vi "Tests_ping.vi"() -> ()   [LabVIEW 2019]
uses:
  <vilib>/Platform/TimedLoop/XDataNode/timing_clust.ctl
  <vilib>/Platform/TimedLoop/XDataNode/nitl_modes.ctl
  <vilib>/Platform/TimedLoop/XDataNode/wakeup.ctl
  <vilib>/Utility/file.llb/Read Delimited Spreadsheet (string).vi
  <vilib>/Platform/TimedLoop/XDataNode/XDataNode.xnode
  <vilib>/Platform/TimedLoop/XDataNode/XDNodeRunTimeDep.lvlib
panel:
  in  "Bouton OK":bool
  out "Booléen":bool
  in  "stop":bool
  out "Systèmes inatteignable":string[][](array[string])
  out "Status":i32(ring) items=["Success"=0, "DestinationNetworkUnreachable"=11002, "DestinationHostUnreachable"=11003, "DestinationProhibited, DestinationProtocolUnreachable"=11004, "DestinationPortUnreachable"=11005, "NoResources"=11006, "BadOption"=11007, "HardwareError"=11008, "PacketTooBig"=11009, "TimedOut"=11010, "BadRoute"=11012, "TtlExpired"=11013, "TtlReassemblyTimeExceeded"=11014, "ParameterProblem"=11015, "SourceQuench"=11016, "BadDestination"=11018, "DestinationUnreachable"=11040, "TimeExceeded"=11041, "BadHeader"=11042, "UnrecognizedNextHeader"=11043, "IcmpError"=11044, "DestinationScopeMismatch"=11045, "Unknown"=-1]
  out "all rows":string[][](array[string]) caption="toutes les lignes"
  # "Tests réseau"
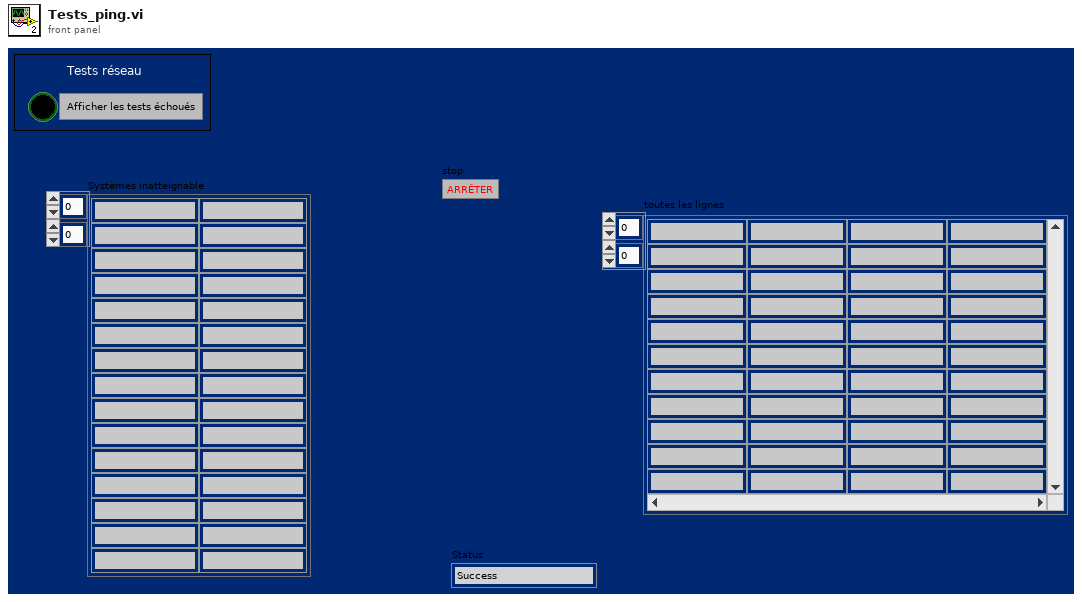
[diagram p1: front panel]
types:
  T1 = typedef "XDNodeRunTimeDep.lvlib/timing_clust.ctl" = cluster{"Expected End [f-1]":u64, "Actual End [f-1]":u64, "Finished Late? [f-1]":bool, "Expected End [i-1]":u64, "Actual End [i-1]":u64, "Finished Late? [i-1]":bool, "Expected Start [i]":u64, "Actual Start [i]":u64, "Expected Start [f]":u64, "Actual Start [f]":u64, "Source Name":string, "Structure Name":string, "Period":i64, "Deadline":i64, "Offset":i64, "Start":i64, "Priority":i32, "Timeout":i32, "Mode":T2, "Wakeup Reason":T3, "Error":errorcluster, "Source Type":string, "Secondary Source Type":string, "Global End Time":u64, "Global Start Time":u64, "Frame Duration":u64, "Iteration Duration":u64, "Assigned CPU":i32, "I/O Scan Engine Mode":u32}
  T2 = typedef "XDNodeRunTimeDep.lvlib/nitl_modes.ctl" = enum32{"No Change", "Process missed periods, maintain original phase", "Discard missed periods, maintain original phase", "Process missed periods, ignore original phase", "Discard missed periods, ignore original phase"}
  T3 = typedef "XDNodeRunTimeDep.lvlib/wakeup.ctl" = enum32{"Normal", "Aborted", "Asynchronous wakeup", "Timing source error", "Timed loop error", "Timeout"}
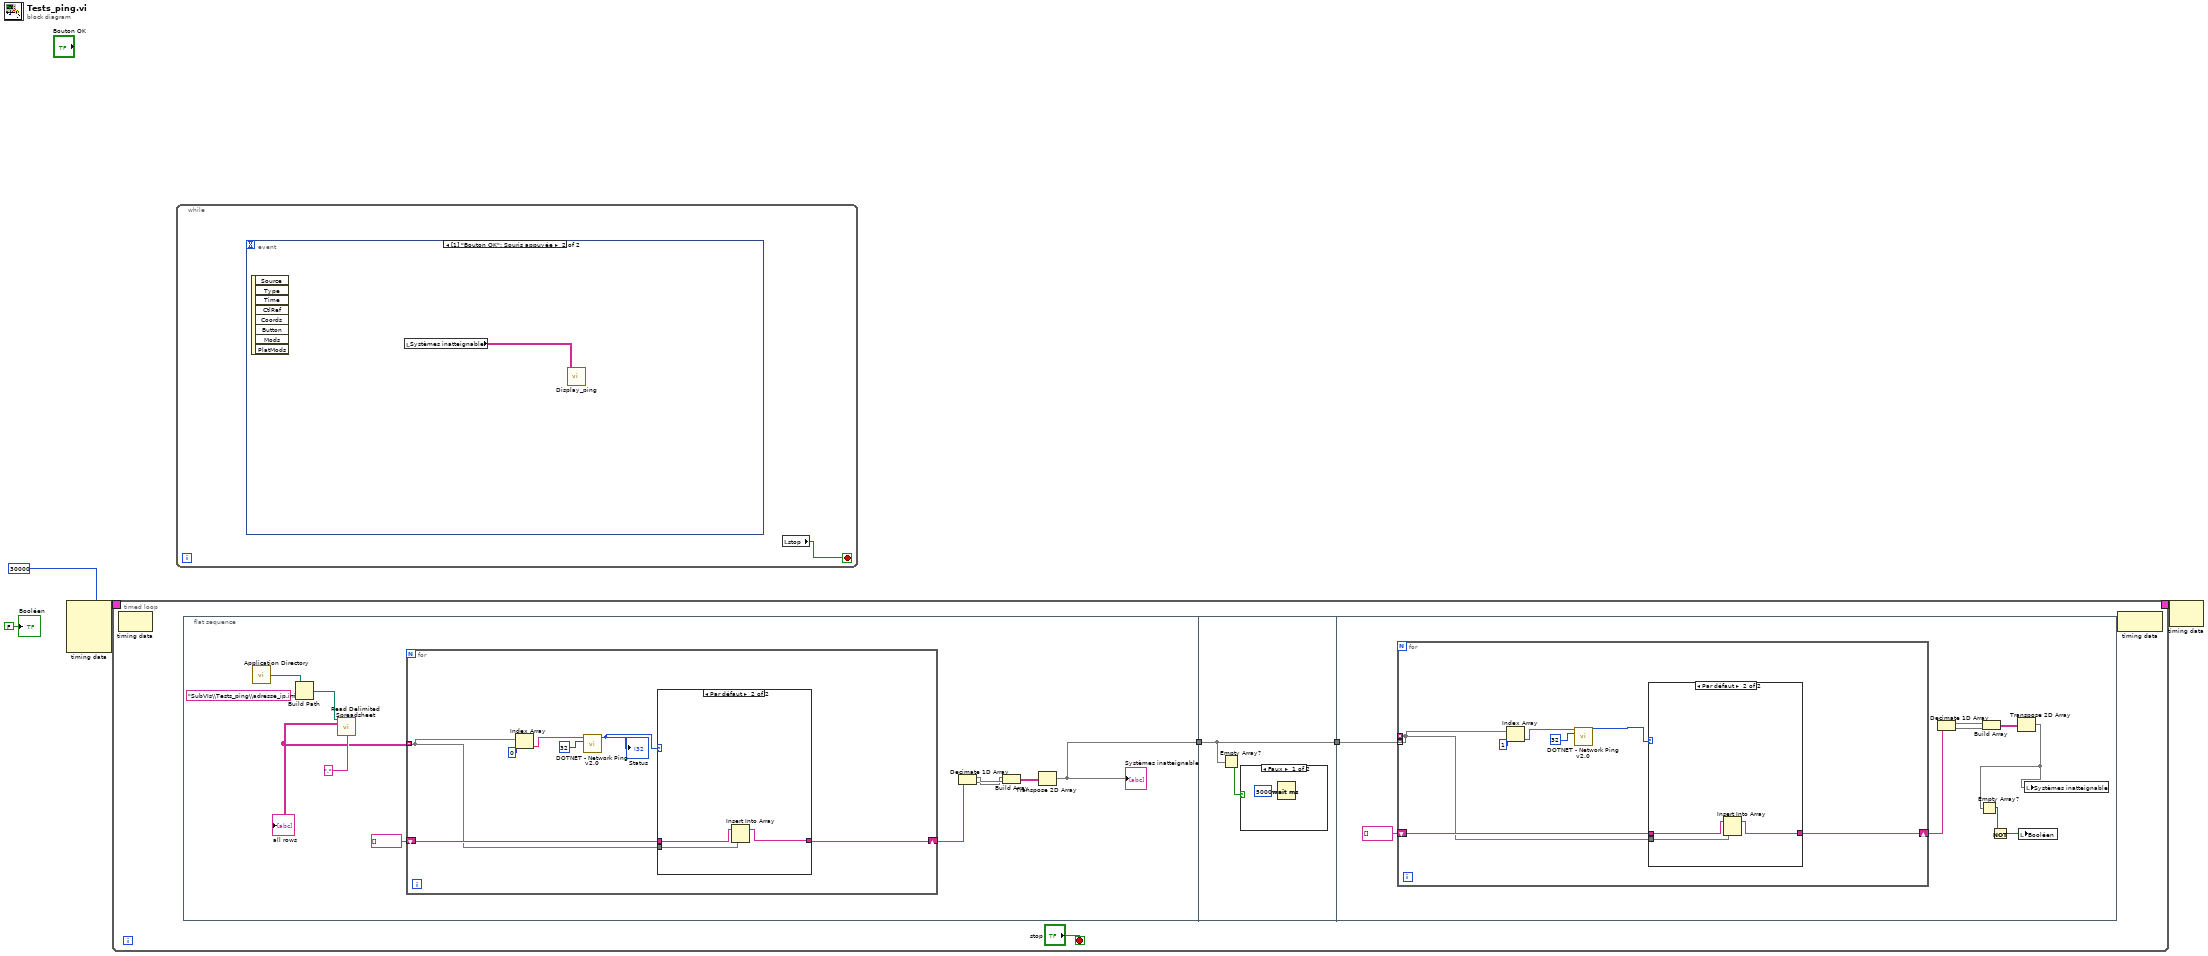
[diagram p0: block diagram]
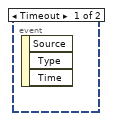
[diagram p2: hidden frame]
diagram:
  n1 = node-c288(i64 30000 ("Période")) -> (w4:T1)  [unwired: 3 in]
  n2 = timed-loop {
    timing: w4 -> [_]
    timing-out: [_] -> w3
    stop <- "stop" stop-if-true
    n3 = node-c288() -> ()  [unwired: 1 in, 1 out]
    n4 = flat-sequence {
      tunnel: [w10] -> w6
      tunnel: w6 -> [w30]
      tunnel: [w30] -> w5
      tunnel: w5 -> [w41]
      frame #0 {
        n5 = call <vilib>:"Application Directory.vi"() -> ("Application Directory"=w17:path)
        n6 = Build Path(base path=w17, name or relative path="SubVIs\\Tests_ping\\adresse_ip.ini" ("nom ou chemin relatif")) -> (appended path=w15:path)
        n7 = call-poly <vilib>:"Read Delimited Spreadsheet.vi"("file path (dialog if empty)"=w15, "delimiter (\\t)"="," ("delimiter (\\t)")) -> ("all rows"=w14:string[][])  [unwired: 8 in, 5 out]
        "all rows" <- w14
        n8 = for {
          tunnel: w14 -> [w19] mode=indexing
          shift-right: [w21] -> w13
          shift-left: string[] [] -> [w20]
          n9 = Index Array(array=w19, index=0 ("indice")) -> (element=w24:string)
          n10 = call "DOTNET - Network Ping v2.0.vi"("IP/Address"=w24, "SetSize"=32) -> ("Status"=w22:i32)  [unwired: 11 in, 2 out]
          "Status" <- w22
          n11 = case shown="Par défaut" w22 {
            tunnel: [w26 w29] -> w21
            tunnel: w20 -> [w26 w28]
            tunnel: w19 -> [_ w27]
            frame 0 {
            }
            frame Default {
              n12 = Insert Into Array(array=w28, new element=w27) -> (w29:string[])  [unwired: 1 in]
            }
          }
        }
        n13 = Decimate 1D Array(w13) -> (w9:string[], w8:string[])
        n14 = Build Array(w8, w9) -> (w12:string[][])
        n15 = Transpose 2D Array(2D array=w12) -> (transposed array=w10:string[][])
        "Systèmes inatteignable" <- w10
      }
      frame #1 {
        n16 = Empty Array?(array=w30) -> (empty?=w31:bool)
        n17 = case shown="Faux" w31 {
          frame False {
            n18 = Wait (ms)(milliseconds to wait=u32 5000 ("attente (ms)")) -> ()  [unwired: 1 out]
          }
          frame True {
          }
        }
      }
      frame #2 {
        n19 = for {
          tunnel: [w43] -> _ mode=indexing
          shift-right: [w42] -> w39
          shift-left: string[] [] -> [w44]
          tunnel: w41 -> [w43] mode=indexing
          n20 = Index Array(array=w43, index=1 ("indice")) -> (element=w47:string)
          n21 = call "DOTNET - Network Ping v2.0.vi"("IP/Address"=w47, "SetSize"=32) -> ("Status"=w45:i32)  [unwired: 11 in, 2 out]
          n22 = case shown="Par défaut" w45 {
            tunnel: [w49 w52] -> w42
            tunnel: w44 -> [w49 w51]
            tunnel: w43 -> [_ w50]
            frame 0 {
            }
            frame Default {
              n23 = Insert Into Array(array=w51, new element=w50) -> (w52:string[])  [unwired: 1 in]
            }
          }
        }
        n24 = Decimate 1D Array(w39) -> (w34:string[], w33:string[])
        n25 = Build Array(w34, w33) -> (w40:string[][])
        n26 = Transpose 2D Array(2D array=w40) -> (transposed array=w36:string[][])
        n27 = Empty Array?(array=w36) -> (empty?=w38:bool)
        n28 = Not(x=w38) -> (.not. x?=w37:bool)
        n29 = local write "Booléen"(w37) -> ()
        n30 = local write "Systèmes inatteignable"(w36) -> ()
      }
    }
    n31 = node-c288() -> ()  [unwired: 1 in, 1 out]
  }
  n32 = while {
    stop <- w55 stop-if-true
    n33 = event shown="[1] \"Bouton OK\": Souris appuyée" {
      selector: _ -> [_ _]
      dyn-events: _ -> [_ _]
      timeout: _ -> [_ _]
      event Timeout {
        n34 = event-data() -> ()  [unwired: 1 in, 3 out]
      }
      event "Bouton OK": Mouse Down {
        n35 = event-data() -> ()  [unwired: 1 in, 8 out]
        n36 = local read "Systèmes inatteignable"() -> (w56:string[][])
        n37 = call "Display_ping.vi"("Systèmes inatteignable"=w56) -> ()  [unwired: 11 in]
      }
    }
    n38 = local read "stop"() -> (w55:bool)
  }
  n39 = node-c288(w3) -> ()  [unwired: 1 out]
  "Booléen" <- FALSE ("Booléen")
